vi "AD2andExtAWG_Init.vi"(0 "object in":refnum<class "AD2andExtAWG.lvclass">, 2 "VISA resource name":refnum<visa-resource-name>, 5 "error in (no error)":errorcluster) -> (14 "object out":refnum<class "AD2andExtAWG.lvclass">, 19 "error out":errorcluster)   [LabVIEW 2019, in "AD2andExtAWG.lvclass"]
uses:
  AD2andExtAWG.lvclass
  AD2_SDK_class/AD2_SDK.lvclass
  AFG3022B_class/AFG3022B.lvclass
  C:/GIT/ThermalAcousticProject/AD2_SDK_class/AD2_SDK.lvclass
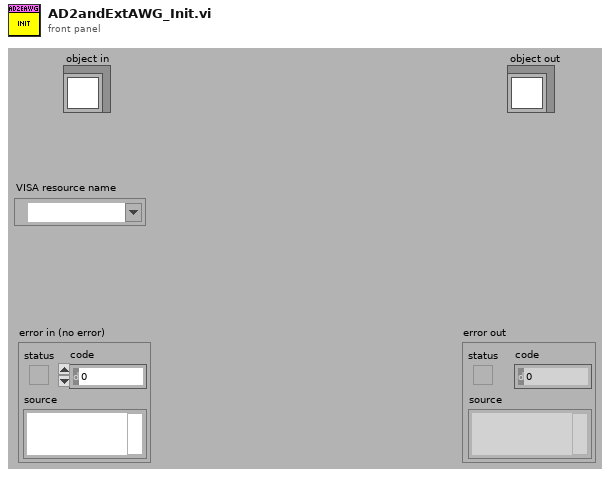
[diagram p1: front panel]
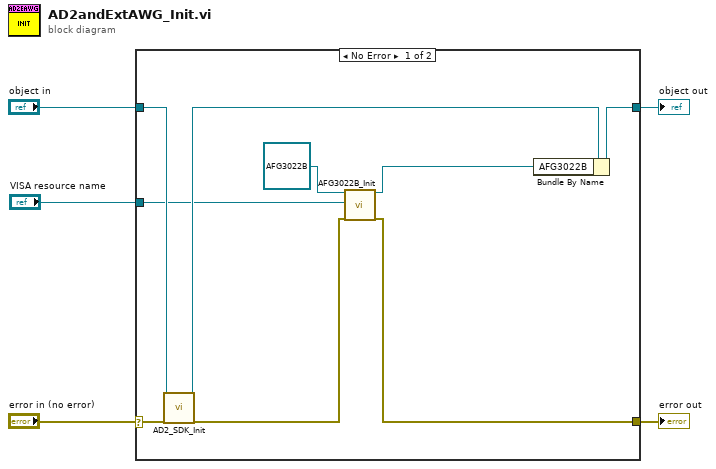
[diagram p0: block diagram]
diagram:
  n1 = case shown="No Error" "error in (no error)" {
    selector: "error in (no error)" -> [w13 w15]
    tunnel: [w14 w16] -> w5
    tunnel: "object in" -> [w12 w16]
    tunnel: [w8 w15] -> w2
    tunnel: "VISA resource name" -> [w7 _]
    frame No Error {
      n2 = call "AD2_SDK_Init.vi"("object in"=w12, "error in (no error)"=w13) -> ("object out"=w11:refnum<class "AD2andExtAWG.lvclass">, "error out"=w9:errorcluster)  [unwired: 16 in]
      n3 = call "AFG3022B_Init.vi"("object in"=refnum<class "AFG3022B.lvclass"> refnum, "VISA resource name"=w7, "error in (no error)"=w9) -> ("object out"=w10:refnum<class "AFG3022B.lvclass">, "error out"=w8:errorcluster)  [unwired: 15 in]
      n4 = Bundle By Name(cluster=w11, "AFG3022B"=w10) -> (w14:refnum<class "AD2andExtAWG.lvclass">)
    }
    frame Error {
    }
  }
  "object out" <- w5
  "error out" <- w2
